vi "TDMS.SplitPropertiesAndChannels.vi"(8 "error in":errorcluster, 11 "Properties":variant) -> (0 "error out":errorcluster, 2 "Properties":variant, 3 "Channels":variant)   [LabVIEW 2015, in "NIAnalysis.lvlib"]
uses:
  NIAnalysis.lvlib
  Types/PropertyGroups.ctl
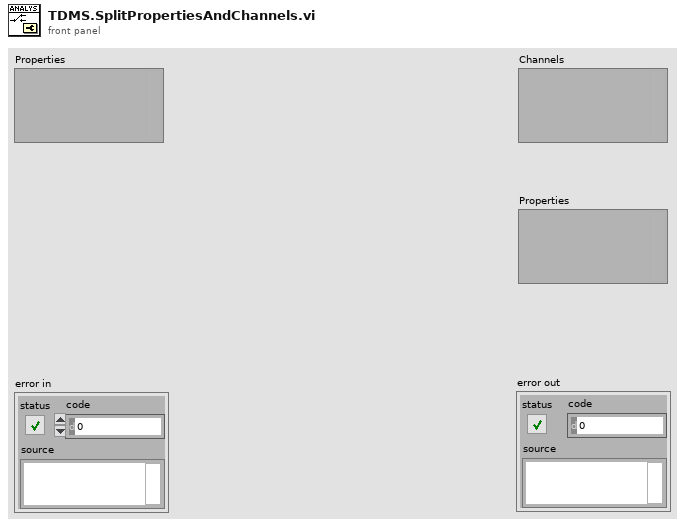
[diagram p1: front panel]
types:
  T1 = typedef "NIAnalysis.lvlib/PropertyGroups.ctl" = cluster{"Pass":bool, "Additional Info":variant}
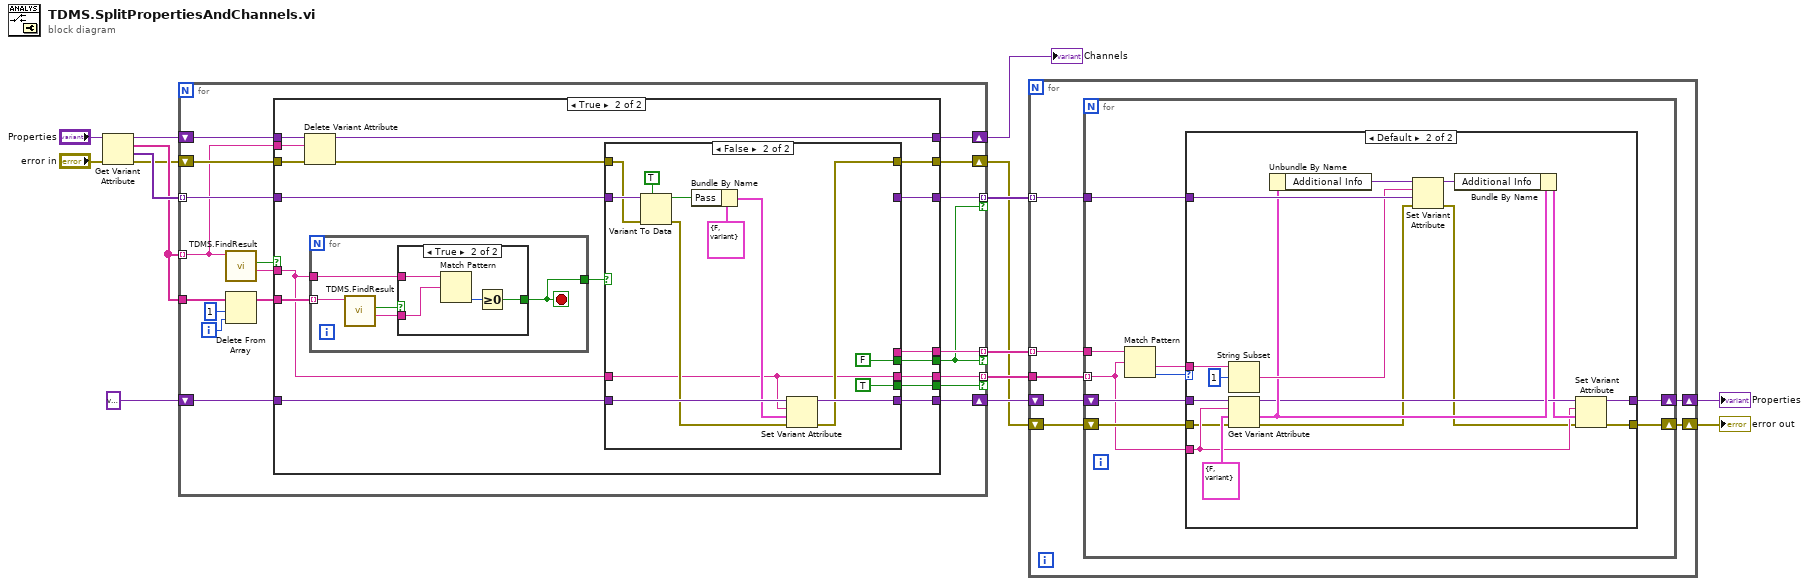
[diagram p0: block diagram]
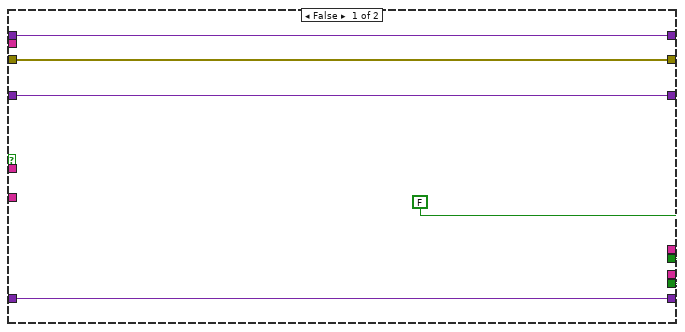
[diagram p3: hidden frame]
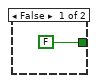
[diagram p4: hidden frame]
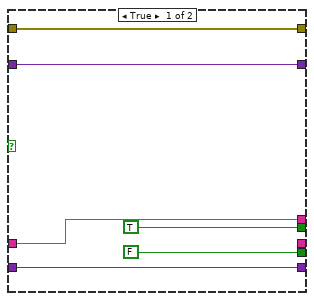
[diagram p5: hidden frame]
diagram:
  n1 = Get Variant Attribute(Variant="Properties", error in="error in") -> (duplicate Variant=w2:variant, names=w6:string[], values=w7:variant[], error out=w4:errorcluster)  [unwired: 2 in]
  n2 = for {
    tunnel: w6 -> [w34]
    tunnel: w6 -> [w17] mode=indexing
    shift-right: [w32] -> w14
    shift-left: variant -> [w33]
    tunnel: w7 -> [w31] mode=indexing
    shift-right: [w30] -> w10
    shift-left: w4 -> [w29]
    tunnel: [w28] -> w13 mode=indexing if=w26
    tunnel: [w27] -> w12 mode=indexing if=w26
    tunnel: [w25] -> w11 mode=indexing if=w24
    shift-right: [w16] -> w1
    shift-left: w2 -> [w18]
    i -> [w19]
    n3 = call "TDMS.FindResult.vi"("Property in"=w17) -> ("Property Text"=w22:string, "Result"=w23:bool)  [unwired: 8 in, 1 out]
    n4 = Delete From Array(array=w34, length=1, index=w19) -> (array with subset deleted=w21:string[])  [unwired: 1 out]
    n5 = case shown="True" w23 {
      tunnel: w21 -> [_ w56]
      tunnel: w33 -> [w35 w55]
      tunnel: [w35 w54] -> w32
      tunnel: w22 -> [_ w52]
      tunnel: w31 -> [w39 w51]
      tunnel: [w37 w50] -> w30
      tunnel: w29 -> [w37 w41]
      tunnel: [_ w49] -> w28
      tunnel: [w39 w48] -> w27
      tunnel: [w38 w47] -> w26
      tunnel: [_ w46] -> w25
      tunnel: [w38 w45] -> w24
      tunnel: w18 -> [w36 w44]
      tunnel: w17 -> [_ w43]
      tunnel: [w36 w42] -> w16
      frame False {
        w38 = FALSE
      }
      frame True {
        n6 = Delete Variant Attribute(4:w41, 6:w43, 7:w44) -> (0:w40:errorcluster, 3:w42:variant)  [unwired: 1 out]
        n7 = for {
          tunnel: w56 -> [w60] mode=indexing
          tunnel: [w57] -> w53
          tunnel: w52 -> [w59]
          stop <- w57 stop-if-true
          n8 = call "TDMS.FindResult.vi"("Property in"=w60) -> ("Property Text"=w58:string, "Result"=w61:bool)  [unwired: 8 in, 1 out]
          n9 = case shown="True" w61 {
            tunnel: w59 -> [_ w65]
            tunnel: w58 -> [_ w64]
            tunnel: [FALSE w63] -> w57
            frame False {
            }
            frame True {
              n10 = Match Pattern(string=w65, regular expression=w64) -> (offset past match=w66:i32)  [unwired: 1 in, 3 out]
              n11 = Greater Or Equal To 0?(x=w66) -> (x >= 0?=w63:bool)
            }
          }
        }
        n12 = case shown="False" w53 {
          tunnel: w55 -> [w71 w85]
          tunnel: [w71 w84] -> w54
          tunnel: w52 -> [w70 w74]
          tunnel: w51 -> [w69 w83]
          tunnel: [w72 w77] -> w50
          tunnel: w40 -> [w72 w76]
          tunnel: [w70 _] -> w49
          tunnel: [w69 _] -> w48
          tunnel: [TRUE FALSE] -> w47
          tunnel: [_ w74] -> w46
          tunnel: [FALSE TRUE] -> w45
          frame True {
          }
          frame False {
            n13 = Variant To Data(error in=w76, type=TRUE, Variant=w83) -> (data=w80:bool, error out=w81:errorcluster)
            n14 = Bundle By Name(cluster=T1 {"Pass"=FALSE, "Additional Info"=variant}, "Pass"=w80) -> (w78:T1)
            n15 = Set Variant Attribute(Variant=w85, name=w74, value=w78, error in=w81) -> (Variant out=w84:variant, error out=w77:errorcluster)  [unwired: 1 out]
          }
        }
      }
    }
  }
  "Channels" <- w1
  n16 = for {
    shift-right: [w87] -> w9
    shift-left: w14 -> [w90]
    tunnel: w13 -> [w92] mode=indexing
    tunnel: w12 -> [w89] mode=indexing
    tunnel: w11 -> [w91]
    shift-right: [w86] -> w8
    shift-left: w10 -> [w88]
    n17 = for {
      tunnel: w92 -> [w93]
      tunnel: w91 -> [w94] mode=indexing
      shift-right: [w98] -> w87
      shift-left: w90 -> [w101]
      tunnel: w89 -> [w100]
      shift-right: [w97] -> w86
      shift-left: w88 -> [w99]
      n18 = Match Pattern(string=w93, regular expression=w94) -> (after substring=w95:string, offset past match=w96:i32)  [unwired: 1 in, 2 out]
      n19 = case shown="Default" w96 {
        tunnel: w94 -> [_ w109]
        tunnel: w101 -> [w103 w120]
        tunnel: w100 -> [_ w117]
        tunnel: w95 -> [_ w116]
        tunnel: w99 -> [w102 w106]
        tunnel: [w103 w105] -> w98
        tunnel: [w102 w104] -> w97
        frame -1 {
        }
        frame Default {
          n20 = String Subset(string=w116, offset (0)=1) -> (substring=w115:string)  [unwired: 1 in]
          n21 = Get Variant Attribute(Variant=w120, name=w109, default value (empty Variant)=T1 {"Pass"=FALSE, "Additional Info"=variant}, error in=w106) -> (duplicate Variant=w111:variant, value=w113:T1, error out=w108:errorcluster)  [unwired: 1 out]
          n22 = Unbundle By Name(w113) -> ("Additional Info"=w118:variant)
          n23 = Set Variant Attribute(Variant=w118, name=w115, value=w117, error in=w108) -> (Variant out=w112:variant, error out=w107:errorcluster)  [unwired: 1 out]
          n24 = Bundle By Name(cluster=w113, "Additional Info"=w112) -> (w110:T1)
          n25 = Set Variant Attribute(Variant=w111, name=w109, value=w110, error in=w107) -> (Variant out=w105:variant, error out=w104:errorcluster)  [unwired: 1 out]
        }
      }
    }
  }
  "Properties" <- w9
  "error out" <- w8
